vi "ACRserverRead.vi"() -> ()   [LabVIEW 2015]
panel:
  out "Read result":dbl
  in  "ComACRServerLib.IChannel":refnum<k7>
  in  "bstrIP Property":string="192.168.10.40"
  out "Connect error out":errorcluster
  in  "Connect error in \n(no error)":errorcluster
  out "Read error out":errorcluster
  in  "Read error in \n(no error)":errorcluster
  in  "ACR P Parameter":string="p38144"
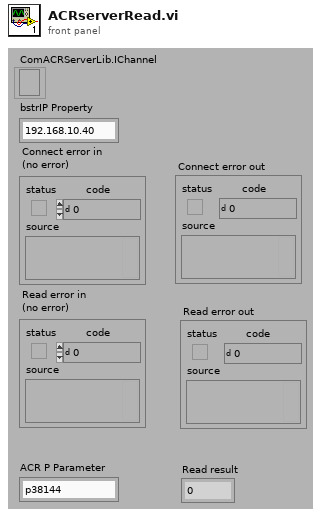
[diagram p1: front panel]
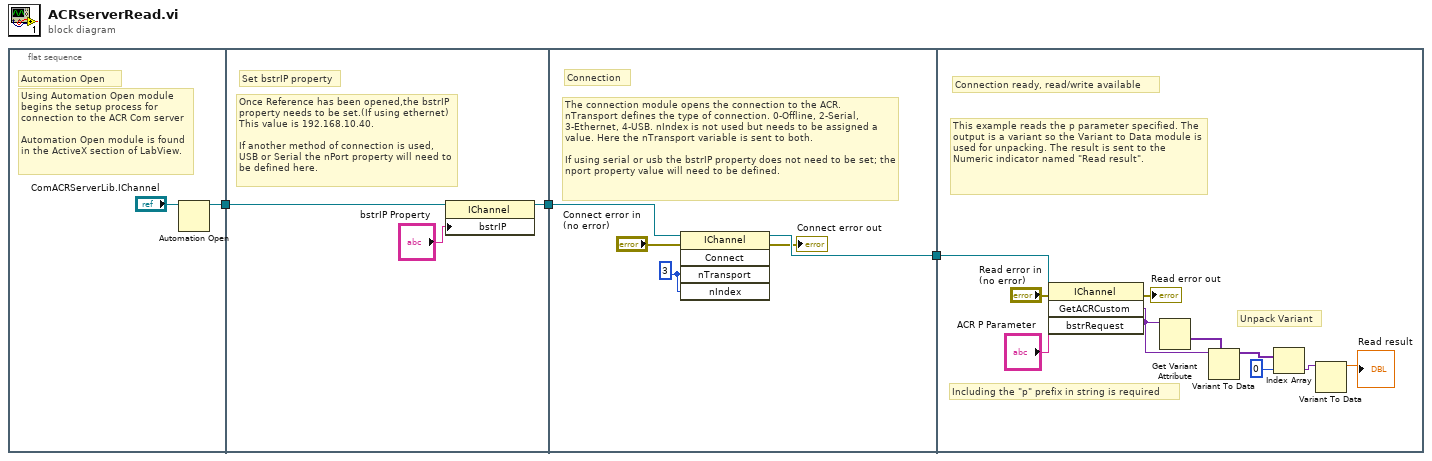
[diagram p0: block diagram]
diagram:
  n1 = flat-sequence {
    tunnel: [w4] -> w1
    tunnel: [w8] -> w2
    tunnel: w1 -> [w6]
    tunnel: [w13] -> w3
    tunnel: w2 -> [w10]
    tunnel: w3 -> [w20]
    frame #0 {
      # "Using Automation Open module begins the setup process for connection to the ACR Com server\n\nAutomation Open module is found\nin the ActiveX section of LabView."
      # "Automation Open"
      n2 = Automation Open(Automation Refnum="ComACRServerLib.IChannel") -> (Automation Refnum=w4:refnum<k7>)  [unwired: 1 in, 3 out]
    }
    frame #1 {
      # "Once Reference has been opened,the bstrIP property needs to be set.(If using ethernet) This value is 192.168.10.40. \n\nIf another method of connection is used, USB or Serial the nPort property will need to be defined here."
      # "Set bstrIP property"
      n3 = property class="IChannel"(reference=w6, "bstrIP"="bstrIP Property") -> (reference out=w8:refnum<k7>)  [unwired: 1 in, 1 out]
    }
    frame #2 {
      w9 = 3
      # "The connection module opens the connection to the ACR. nTransport defines the type of connection. 0-Offline, 2-Serial, 3-Ethernet, 4-USB. nIndex is not used but needs to be assigned a value. Here the nTransport variable is sent to both.\n\nIf using serial or usb the bstrIP property does not need to be set; the nport property value will need to be defined."
      # "Connection"
      n4 = invoke class="IChannel" method="Connect"(reference=w10, error in="Connect error in \n(no error)", "nTransport"=w9, "nIndex"=w9) -> (reference out=w13:refnum<k7>, error out=→"Connect error out":errorcluster)  [unwired: 1 in, 3 out]
    }
    frame #3 {
      # "Including the \"p\" prefix in string is required"
      # "Unpack Variant"
      # "This example reads the p parameter specified. The output is a variant so the Variant to Data module is used for unpacking. The result is sent to the Numeric indicator named \"Read result\"."
      # "Connection ready, read/write available"
      n5 = invoke class="IChannel" method="GetACRCustom"(reference=w20, error in="Read error in \n(no error)", "bstrRequest"="ACR P Parameter") -> (error out=→"Read error out":errorcluster, "GetACRCustom"=w18:variant)  [unwired: 1 in, 2 out]
      n6 = Get Variant Attribute(Variant=w18) -> (values=w19:variant[])  [unwired: 1 in, 5 out]
      n7 = Variant To Data(type=w19, Variant=w18) -> (data=w17:variant[])  [unwired: 1 in, 1 out]
      n8 = Index Array(array=w17, index=0) -> (element=w15:variant)
      n9 = Variant To Data(Variant=w15) -> (data=→"Read result":dbl)  [unwired: 2 in, 1 out]
    }
  }
